vi "onStarted.vi"(8 "error in (no error)":errorcluster, 11 "demoForJoe":refnum<class "demoForJoe.lvclass">) -> (0 "error out":errorcluster, 3 "demoForJoe out":refnum<class "demoForJoe.lvclass">)   [LabVIEW 2016, in "demoForJoe.lvclass"]
doc: "JKI State Machine Objects (SMO) 1.2.1.55\nJKI - JKI\nCopyright (c) 2017, JKI"
uses:
  demoForJoe.lvclass
  Typedefs/PrivateEvents--demoForJoe.StringMethod.ctl
  <vilib>/JKI/JKI SMO/SMO/SMO.lvclass
panel:
  # "For instructions on how to use the JKI State Machine Objects, examples and video tutorials, visit:\nhttp://jki.net/state-machine-objects/\n\nJKI State Machine Objects™\nhttp://jki.net/state-machine-objects/\nCopyright (C) 2005-2015, JKI <info@jki.net>\nALL RIGHTS RESERVED"
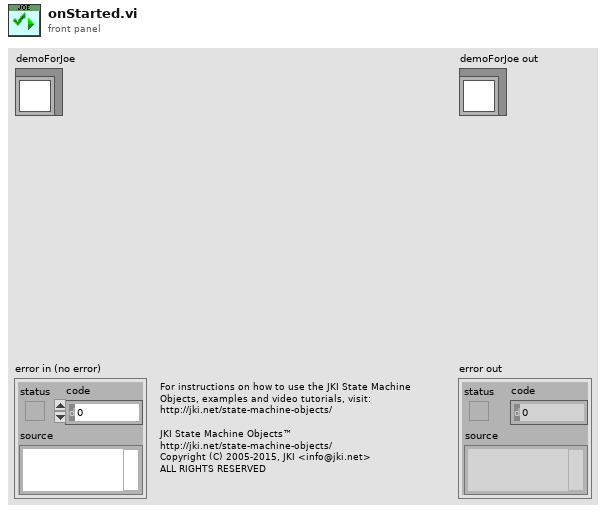
[diagram p1: front panel]
types:
  T1 = typedef "demoForJoe.lvclass/PrivateEvents--demoForJoe.StringMethod.ctl" = string
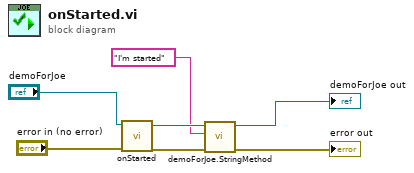
[diagram p0: block diagram]
diagram:
  n1 = call-parent "onStarted.vi"("error in (no error)"="error in (no error)", "SMO"="demoForJoe") -> ("error out"=w4:errorcluster, "SMO out"=w5:refnum<class "demoForJoe.lvclass">)  [unwired: 8 in]
  n2 = call "demoForJoe.StringMethod.vi"("error in (no error)"=w4, "StringMethod"=T1 "I'm started", "demoForJoe"=w5) -> ("error out"=→"error out":errorcluster, "demoForJoe out"=→"demoForJoe out":refnum<class "demoForJoe.lvclass">)  [unwired: 7 in]
